vi "Composition1_Main.vi"() -> (0 "error out":errorcluster)   [LabVIEW 2020]
uses:
  MenuItem_class/MenuItem.lvclass
  C:/Projects/DesignPatterns/Composition/MenuComponent_class/MenuComponent.lvclass
  Menu_class/Menu.lvclass
  Console_class/Console.lvclass
panel:
  out "TextOut":string
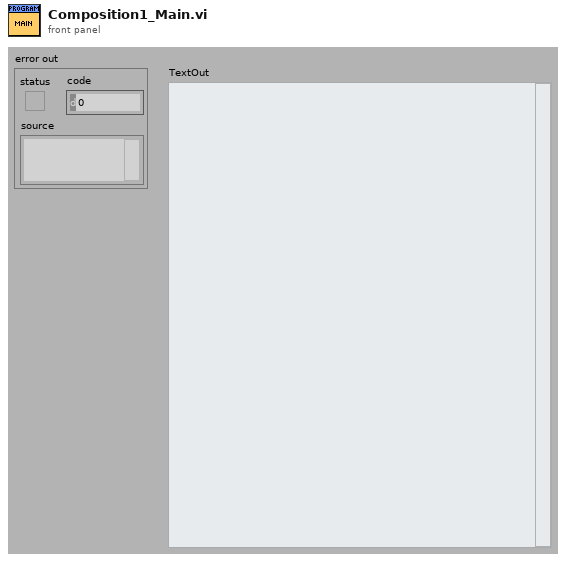
[diagram p1: front panel]
types:
  T1 = cluster{"Name":string, "Name 2":string, "Price":dbl, "Isveg":bool}[]
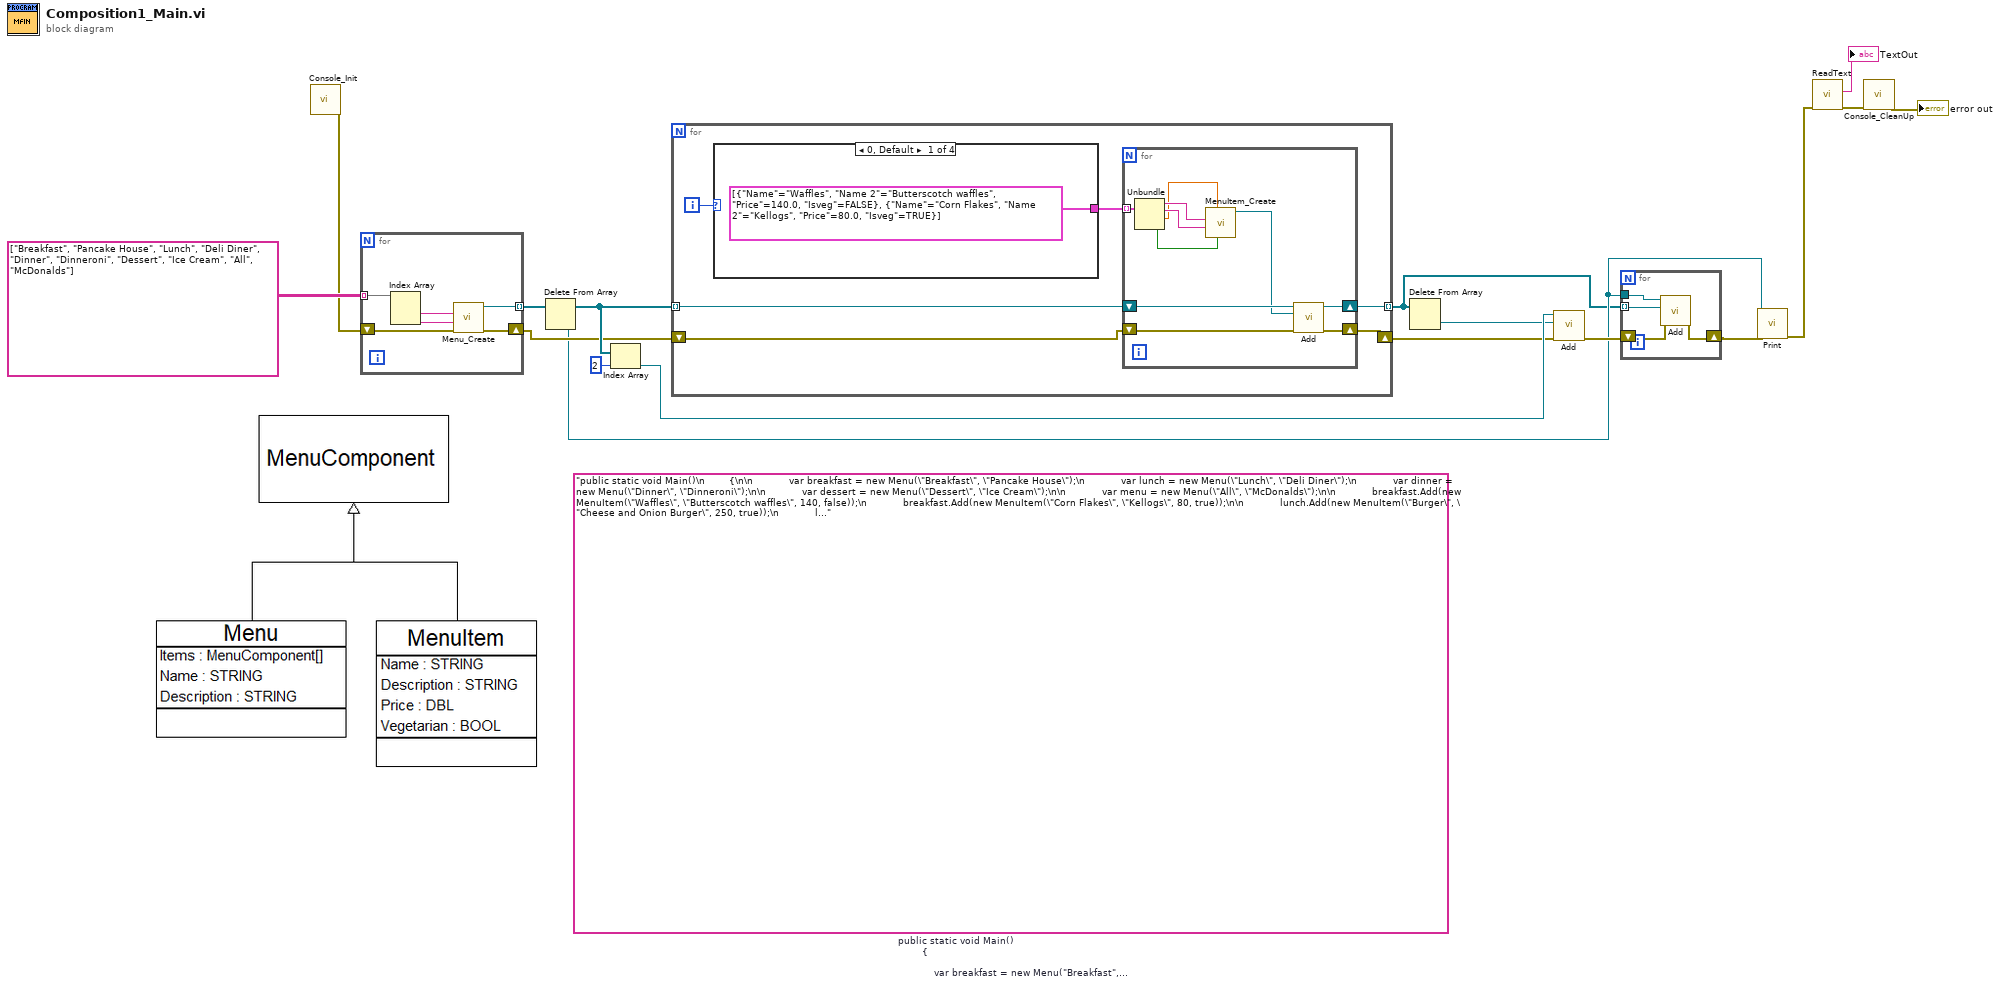
[diagram p0: block diagram]
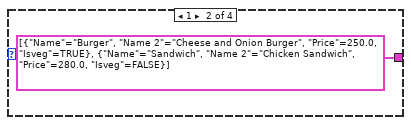
[diagram p2: hidden frame]
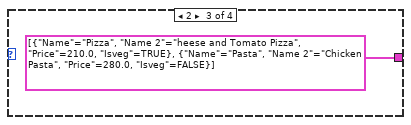
[diagram p3: hidden frame]
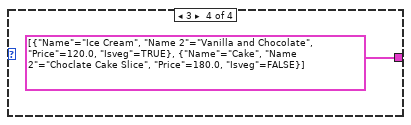
[diagram p4: hidden frame]
diagram:
  (unwired) "public static void Main()\n        {\n\n            var breakfast = new Menu(\"Breakfast\", \"Pancake House\");\n            var lunch = new Menu(\"Lunch\", \"Deli Diner\");\n            var dinner = new Menu(\"Dinner\", \"Dinneroni\");\n\n            var dessert = new Menu(\"Dessert\", \"Ice Cream\");\n\n            var menu = new Menu(\"All\", \"McDonalds\");\n\n            breakfast.Add(new MenuItem(\"Waffles\", \"Butterscotch waffles\", 140, false));\n            breakfast.Add(new MenuItem(\"Corn Flakes\", \"Kellogs\", 80, true));\n\n            lunch.Add(new MenuItem(\"Burger\", \"Cheese and Onion Burger\", 250, true));\n            lunch.Add(new MenuItem(\"Sandwich\", \"Chicken Sandwich\", 280, false));\n\n            dinner.Add(new MenuItem(\"Pizza\", \"Cheese and Tomato Pizza\", 210, true));\n            dinner.Add(new MenuItem(\"Pasta\", \"Chicken Pasta\", 280, false));\n\n            dessert.Add(new MenuItem(\"Ice Cream\", \"Vanilla and Chocolate\", 120, true));\n            dessert.Add(new MenuItem(\"Cake\", \"Choclate Cake Slice\", 180, false));\n\n            dinner.Add(dessert);\n            menu.Add(breakfast);\n            menu.Add(lunch);\n            menu.Add(dinner);\n\n            menu.Print();\n\n        }"  # public static void Main()         {              var breakfast = new Menu("Breakfast", "Pancake House");             var lunch = new Menu("Lunch", "Deli Diner");             var dinner = new Menu("Dinner", "Dinneroni");              var dessert = new Menu("Dessert", "Ice Cream");              var menu = new Menu("All", "McDonalds");              breakfast.Add(new MenuItem("Waffles", "Butterscotch waffles", 140, false));             breakfast.Add(new MenuItem("Corn Flakes", "Kellogs", 80, true));              lunch.Add(new MenuItem("Burger", "Cheese and Onion Burger", 250, true));             lunch.Add(new MenuItem("Sandwich", "Chicken Sandwich", 280, false));              dinner.Add(new MenuItem("Pizza", "Cheese and Tomato Pizza", 210, true));             dinner.Add(new MenuItem("Pasta", "Chicken Pasta", 280, false));              dessert.Add(new MenuItem("Ice Cream", "Vanilla and Chocolate", 120, true));             dessert.Add(new MenuItem("Cake", "Choclate Cake Slice", 180, false));              dinner.Add(dessert);             menu.Add(breakfast);             menu.Add(lunch);             menu.Add(dinner);              menu.Print();          }
  n1 = call "Console_Init.vi"() -> ("Error Out"=w6:errorcluster)  [unwired: 10 in, 1 out]
  n2 = for {
    tunnel: string[][] [["Breakfast", "Pancake House"], ["Lunch", "Deli Diner"], ["Dinner", "Dinneroni"], ["Dessert", "Ice Cream"], ["All", "McDonalds"]] ("Name") -> [w23] mode=indexing
    tunnel: [w20] -> w16 mode=indexing
    shift-right: [w19] -> w9
    shift-left: w6 -> [w18]
    n3 = Index Array(array=w23) -> (element #1=w22:string, element #2=w21:string)  [unwired: 2 in]
    n4 = call "Menu_Create.vi"("Error In"=w18, "Description"=w21, "Name"=w22) -> ("Error Out"=w19:errorcluster, "reference out"=w20:refnum<class "Menu.lvclass">)  [unwired: 7 in]
  }
  n5 = Delete From Array(array=w16) -> (deleted portion=w7:refnum<class "Menu.lvclass">, array with subset deleted=w15:refnum<class "Menu.lvclass">[])  [unwired: 2 in]
  n6 = Index Array(array=w15, index=2) -> (element=w13:refnum<class "Menu.lvclass">)
  n7 = for {
    tunnel: w15 -> [w28] mode=indexing
    tunnel: [w26] -> w1 mode=indexing
    shift-right: [w25] -> w10
    shift-left: w9 -> [w24]
    i -> [w27]
    n8 = case shown="0, Default" w27 {
      tunnel: [T1 [{"Name"="Waffles", "Name 2"="Butterscotch waffles", "Price"=140.0, "Isveg"=FALSE}, {"Name"="Corn Flakes", "Name 2"="Kellogs", "Price"=80.0, "Isveg"=TRUE}] ("Name") T1 [{"Name"="Burger", "Name 2"="Cheese and Onion Burger", "Price"=250.0, "Isveg"=TRUE}, {"Name"="Sandwich", "Name 2"="Chicken Sandwich", "Price"=280.0, "Isveg"=FALSE}] ("Name") T1 [{"Name"="Pizza", "Name 2"="heese and Tomato Pizza", "Price"=210.0, "Isveg"=TRUE}, {"Name"="Pasta", "Name 2"="Chicken Pasta", "Price"=280.0, "Isveg"=FALSE}] ("Name") T1 [{"Name"="Ice Cream", "Name 2"="Vanilla and Chocolate", "Price"=120.0, "Isveg"=TRUE}, {"Name"="Cake", "Name 2"="Choclate Cake Slice", "Price"=180.0, "Isveg"=FALSE}] ("Name")] -> w29
      frame 0, Default {
      }
      frame 1 {
      }
      frame 2 {
      }
      frame 3 {
      }
    }
    n9 = for {
      tunnel: w29 -> [w42] mode=indexing
      shift-right: [w36] -> w26
      shift-left: w28 -> [w43]
      shift-right: [w35] -> w25
      shift-left: w24 -> [w34]
      n10 = Unbundle(w42) -> ("Name"=w41:string, "Name 2"=w40:string, "Price"=w38:dbl, "Isveg"=w39:bool)
      n11 = call "MenuItem_Create.vi"("Isveg"=w39, "Price"=w38, "Description"=w40, "Name"=w41) -> ("reference out"=w37:refnum<class "MenuItem.lvclass">)  [unwired: 6 in, 1 out]
      n12 = call-dynamic "Add.vi"("Error In"=w34, "Component"=w37, "reference in"=w43) -> ("Error Out"=w35:errorcluster, "reference in"=w36:refnum<class "Menu.lvclass">)  [unwired: 7 in]
    }
  }
  n13 = Delete From Array(array=w1) -> (deleted portion=w12:refnum<class "Menu.lvclass">)  [unwired: 2 in, 1 out]
  n14 = call-dynamic "Add.vi"("Error In"=w10, "Component"=w12, "reference in"=w13) -> ("Error Out"=w11:errorcluster)  [unwired: 7 in, 1 out]
  n15 = for {
    tunnel: w7 -> [w47]
    tunnel: w1 -> [w46] mode=indexing
    shift-right: [w44] -> w8
    shift-left: w11 -> [w45]
    n16 = call-dynamic "Add.vi"("Error In"=w45, "Component"=w46, "reference in"=w47) -> ("Error Out"=w44:errorcluster)  [unwired: 7 in, 1 out]
  }
  n17 = call-dynamic "Print.vi"("Error In"=w8, "reference in"=w7) -> ("Error Out"=w5:errorcluster)  [unwired: 8 in, 1 out]
  n18 = call "ReadText.vi"("Error In"=w5) -> ("Error Out"=w3:errorcluster, "TextOut"=→"TextOut":string)  [unwired: 9 in]
  n19 = call "Console_CleanUp.vi"("Error In"=w3) -> ("Error Out"=→"error out":errorcluster)  [unwired: 10 in]
